vi "Initialize.vi"() -> (0 "SmartScope out":refnum<k24>)   [LabVIEW 2015]
uses:
  C:/LabNation/SmartScopeApp/SmartScope/bin/Windows/AnyCPU/Debug/LabNation.DeviceInterface.dll
  LabNation/SmartScopeApp/SmartScope/bin/Windows/AnyCPU/Debug/LabNation.DeviceInterface.dll
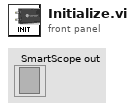
[diagram p1: front panel]
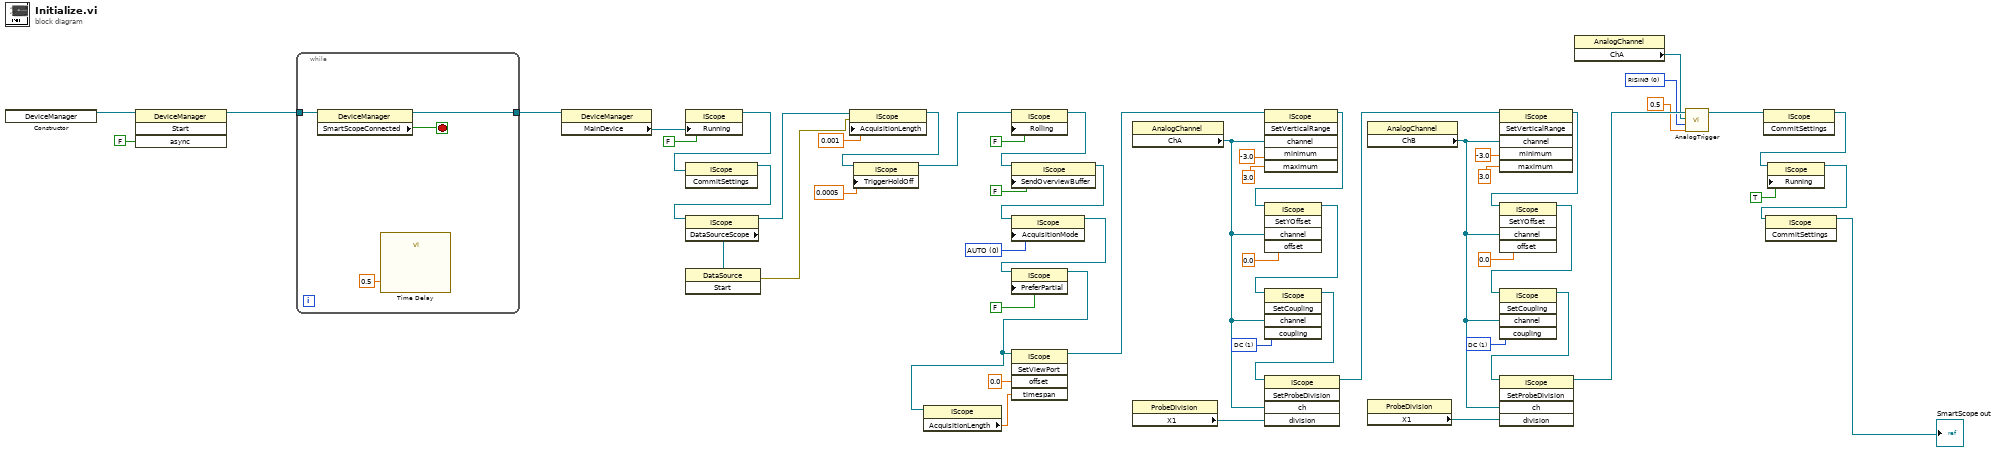
[diagram p0: block diagram]
diagram:
  w43 = 0 items=["RISING", "FALLING", "ANY"] ("edge")
  w37 = 1 items=["AC", "DC"] ("coupling")
  w28 = 1 items=["AC", "DC"] ("coupling")
  w19 = 0 items=["AUTO", "NORMAL", "SINGLE"] ("AcquisitionMode")
  n1 = constructor class="DeviceManager"() -> (reference out=w1:refnum<k24>)  [unwired: 3 in, 2 out]
  n2 = invoke class="DeviceManager" method="Start"(reference=w1, "async"=FALSE) -> (reference out=w2:refnum<k24>)  [unwired: 2 in, 3 out]
  n3 = while {
    tunnel: w2 -> [w57]
    tunnel: [w56] -> w4
    stop <- w55 stop-if-true
    n4 = property class="DeviceManager"(reference=w57) -> (reference out=w56:refnum<k24>, "SmartScopeConnected"=w55:bool)  [unwired: 1 in, 1 out]
    n5 = call "Time Delay"("Delay Time (s)"=0.5) -> ()  [unwired: 10 in, 1 out]
  }
  n6 = property class="DeviceManager"(reference=w4) -> ("MainDevice"=w5:refnum<k24>)  [unwired: 1 in, 2 out]
  n7 = property class="IScope"(reference=w5, "Running"=FALSE) -> (reference out=w7:refnum<k24>)  [unwired: 1 in, 1 out]
  n8 = invoke class="IScope" method="CommitSettings"(reference=w7) -> (reference out=w15:refnum<k24>)  [unwired: 2 in, 2 out]
  n9 = property class="IScope"(reference=w15) -> (reference out=w52:refnum<k24>, "DataSourceScope"=w16:refnum<k24>)  [unwired: 1 in, 1 out]
  n10 = invoke class="DataSource" method="Start"(reference=w16) -> (error out=w48:errorcluster)  [unwired: 2 in, 2 out]
  n11 = property class="IScope"(reference=w52, error in=w48, "AcquisitionLength"=0.001) -> (reference out=w10:refnum<k24>)  [unwired: 1 out]
  n12 = property class="IScope"(reference=w10, "TriggerHoldOff"=0.0005 ("AcquisitionLength")) -> (reference out=w11:refnum<k24>)  [unwired: 1 in, 1 out]
  n13 = property class="IScope"(reference=w11, "Rolling"=FALSE ("LogicAnalyserEnabled")) -> (reference out=w12:refnum<k24>)  [unwired: 1 in, 1 out]
  n14 = property class="IScope"(reference=w12, "SendOverviewBuffer"=FALSE) -> (reference out=w13:refnum<k24>)  [unwired: 1 in, 1 out]
  n15 = property class="IScope"(reference=w13, "AcquisitionMode"=w19) -> (reference out=w14:refnum<k24>)  [unwired: 1 in, 1 out]
  n16 = property class="IScope"(reference=w14, "PreferPartial"=FALSE) -> (reference out=w22:refnum<k24>)  [unwired: 1 in, 1 out]
  n17 = property class="IScope"(reference=w22) -> ("AcquisitionLength"=w23:dbl)  [unwired: 1 in, 2 out]
  n18 = invoke class="IScope" method="SetViewPort"(reference=w22, "offset"=0.0, "timespan"=w23) -> (reference out=w24:refnum<k24>)  [unwired: 2 in, 4 out]
  n19 = property class="AnalogChannel"() -> ("ChA"=w30:refnum<k24>)  [unwired: 2 in, 2 out]
  n20 = property class="ProbeDivision"() -> ("X1"=w31:refnum<k24>)  [unwired: 2 in, 2 out]
  n21 = invoke class="IScope" method="SetVerticalRange"(reference=w24, "channel"=w30, "minimum"=sgl -3.0, "maximum"=sgl 3.0) -> (reference out=w41:refnum<k24>)  [unwired: 2 in, 5 out]
  n22 = invoke class="IScope" method="SetYOffset"(reference=w41, "channel"=w30, "offset"=sgl 0.0) -> (reference out=w53:refnum<k24>)  [unwired: 2 in, 4 out]
  n23 = invoke class="IScope" method="SetCoupling"(reference=w53, "channel"=w30, "coupling"=w28) -> (reference out=w29:refnum<k24>)  [unwired: 2 in, 4 out]
  n24 = invoke class="IScope" method="SetProbeDivision"(reference=w29, "ch"=w30, "division"=w31) -> (reference out=w54:refnum<k24>)  [unwired: 2 in, 4 out]
  n25 = property class="AnalogChannel"() -> ("ChB"=w39:refnum<k24>)  [unwired: 2 in, 2 out]
  n26 = property class="ProbeDivision"() -> ("X1"=w40:refnum<k24>)  [unwired: 2 in, 2 out]
  n27 = invoke class="IScope" method="SetVerticalRange"(reference=w54, "channel"=w39, "minimum"=sgl -3.0, "maximum"=sgl 3.0) -> (reference out=w34:refnum<k24>)  [unwired: 2 in, 5 out]
  n28 = invoke class="IScope" method="SetYOffset"(reference=w34, "channel"=w39, "offset"=sgl 0.0) -> (reference out=w36:refnum<k24>)  [unwired: 2 in, 4 out]
  n29 = invoke class="IScope" method="SetCoupling"(reference=w36, "channel"=w39, "coupling"=w37) -> (reference out=w38:refnum<k24>)  [unwired: 2 in, 4 out]
  n30 = invoke class="IScope" method="SetProbeDivision"(reference=w38, "ch"=w39, "division"=w40) -> (reference out=w50:refnum<k24>)  [unwired: 2 in, 4 out]
  n31 = property class="AnalogChannel"() -> ("ChA"=w42:refnum<k24>)  [unwired: 2 in, 2 out]
  n32 = call "AnalogTrigger.vi"("EdgeType"=sgl 0.5 ("level"), "TriggerLevel"=w43, "AnalogChannel"=w42, "SmartScope in"=w50) -> ("SmartScope out"=w51:refnum<k24>)
  n33 = invoke class="IScope" method="CommitSettings"(reference=w51) -> (reference out=w47:refnum<k24>)  [unwired: 2 in, 2 out]
  n34 = property class="IScope"(reference=w47, "Running"=TRUE) -> (reference out=w46:refnum<k24>)  [unwired: 1 in, 1 out]
  n35 = invoke class="IScope" method="CommitSettings"(reference=w46) -> (reference out=→"SmartScope out":refnum<k24>)  [unwired: 2 in, 2 out]
